vi "BASE-Main.vi"() -> ()   [LabVIEW 2017]
uses:
  <vilib>/Utility/error.llb/DialogType.ctl
  55ed0eea-cd20-493f-8468-85b8c1a0a0c0.vi
  Global/PLC_to_Auto.vi
panel:
  in  "AUTO":bool
  in  "PLAN EDITOR":bool
  in  "UNLOAD":bool
  in  "PLAN CREATOR":bool
  in  "i/o MANUAL":bool
  in  "i/o SCREEN":bool
  in  "HARDWARE SETTING":bool
  out "Status Number":i32
  out "Status":i32(ring)=1 items=["Stopped"=1, "StartPending"=2, "StopPending"=3, "Running"=4, "ContinuePending"=5, "PausePending"=6, "Paused"=7]
  in  "RECIPE":bool
  out "error out":errorcluster
  in  "Logout":bool
  in  "Stop":bool
  in  "Create Login":bool
  in  "Reports":bool
  in  "FEED":bool
  out "Time":string
  out "Date":string
  in  "Login":bool
  # "KITTING STATION"
types:
  T1 = enum8{"Enabled", "Disabled", "Disabled and Grayed Out"}
  T2 = typedef "DialogType.ctl" = u16
  T3 = enum32{"Invalid", "Standard", "Closed", "Hidden", "Minimized", "Maximized"}
  T4 = enum32{"invalid app kind", "Development System", "Run Time System", "Student Edition", "Embedded LabVIEW", "Evaluation", "Custom"}
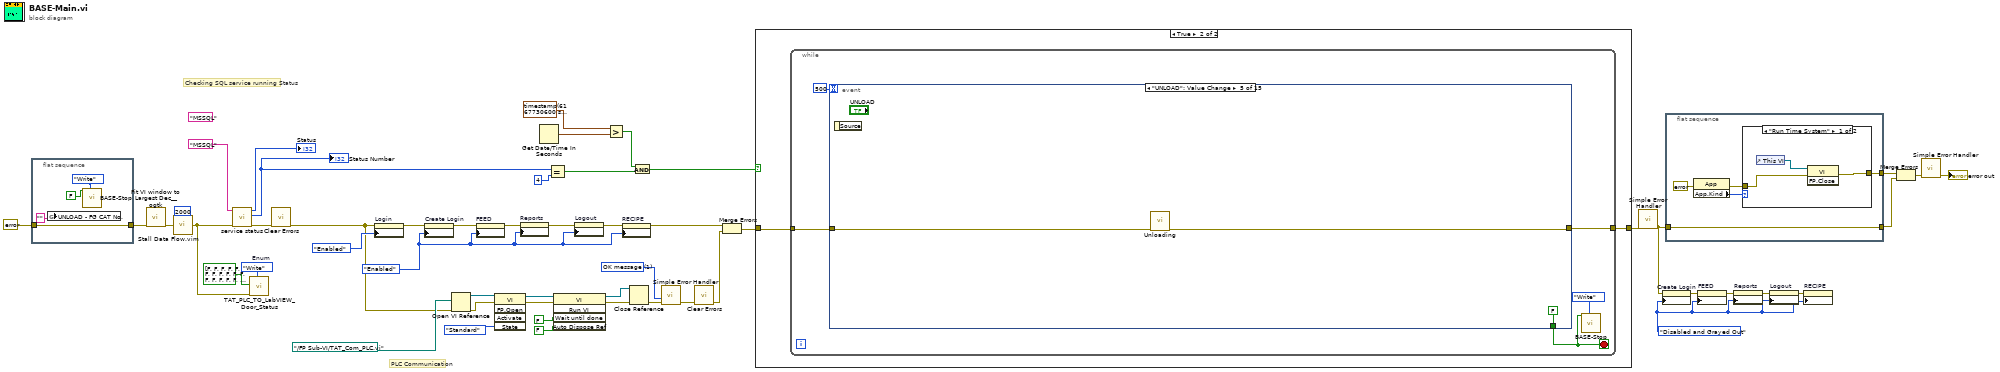
[diagram p0: block diagram]
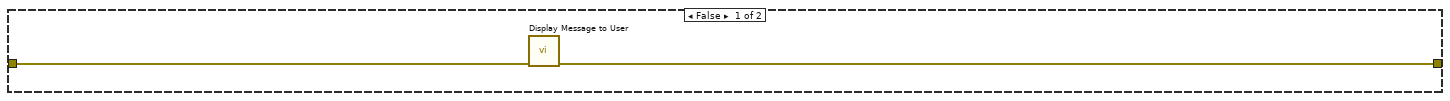
[diagram p3: hidden frame]
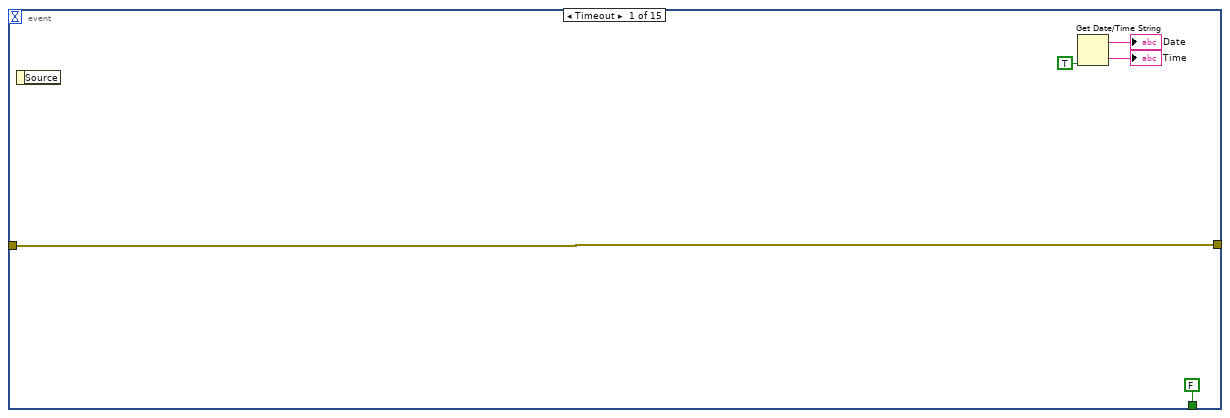
[diagram p4: hidden frame]
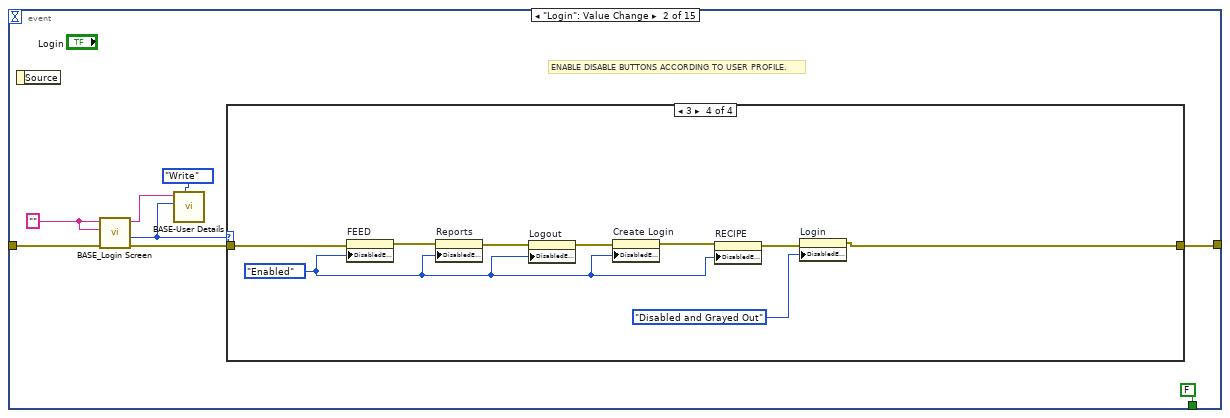
[diagram p5: hidden frame]
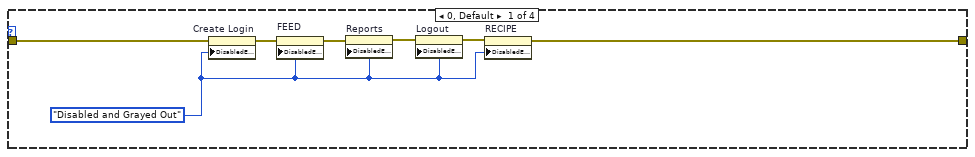
[diagram p6: hidden frame]
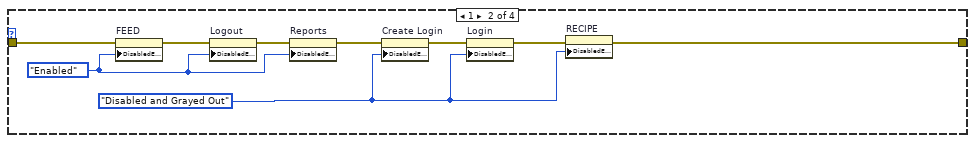
[diagram p7: hidden frame]
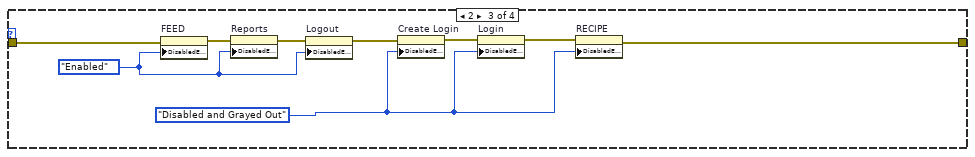
[diagram p8: hidden frame]
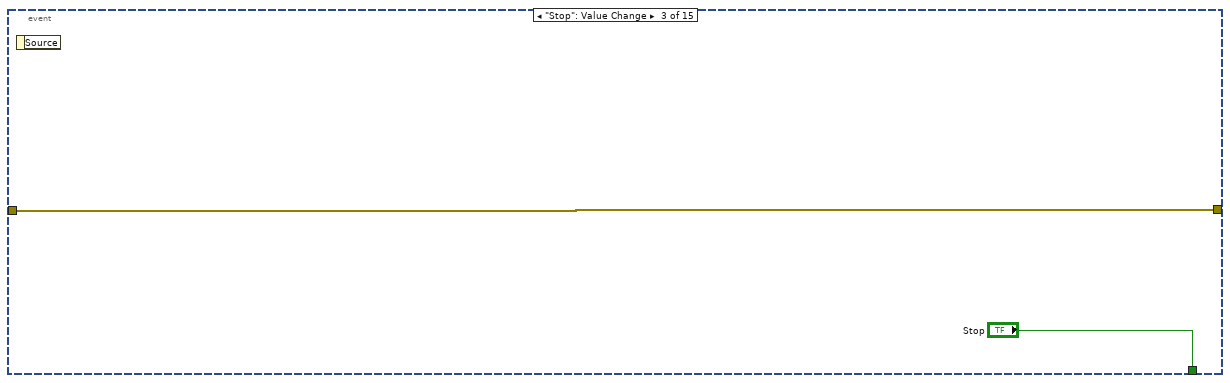
[diagram p9: hidden frame]
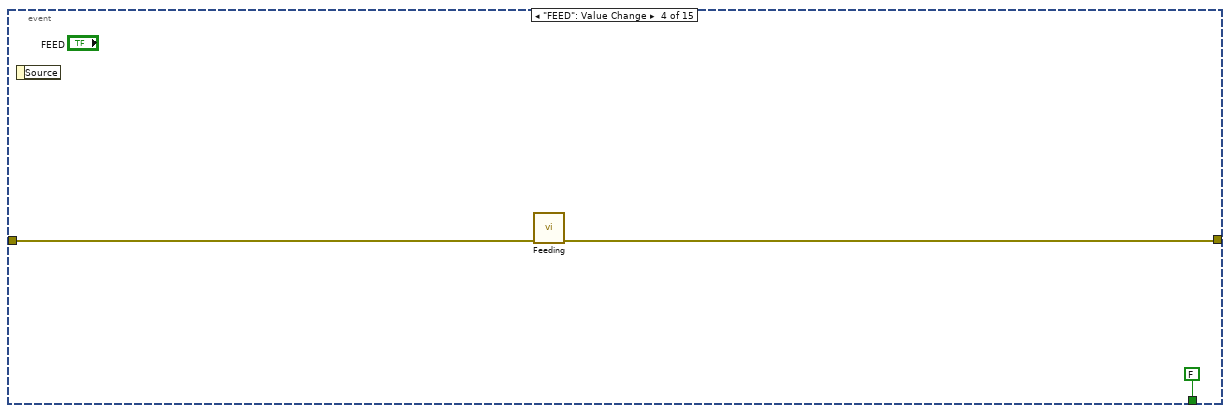
[diagram p10: hidden frame]
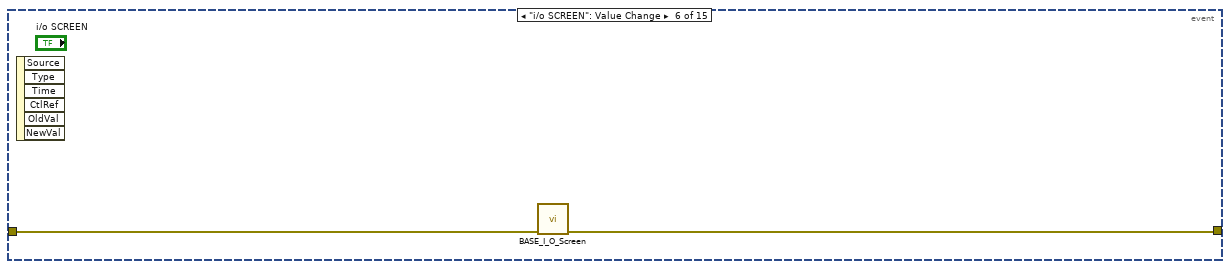
[diagram p11: hidden frame]
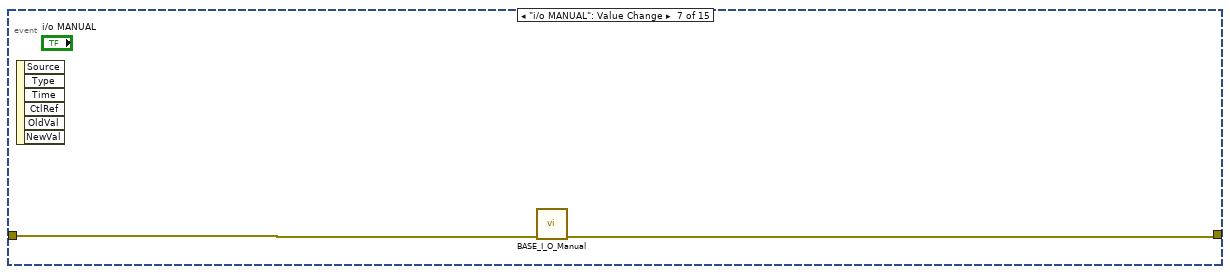
[diagram p12: hidden frame]
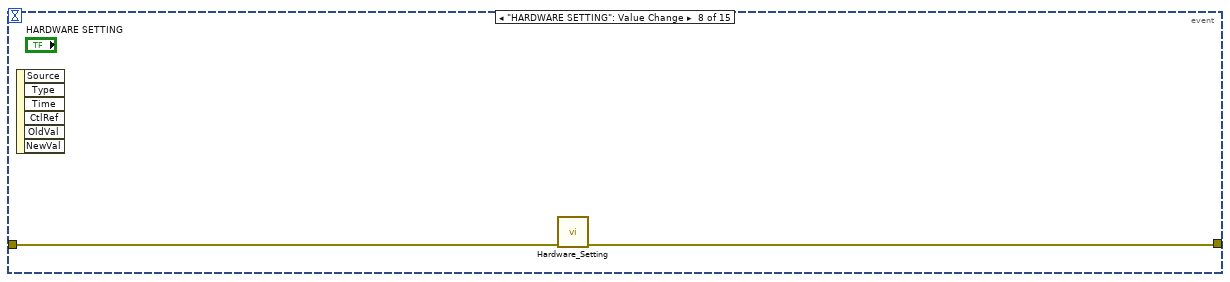
[diagram p13: hidden frame]
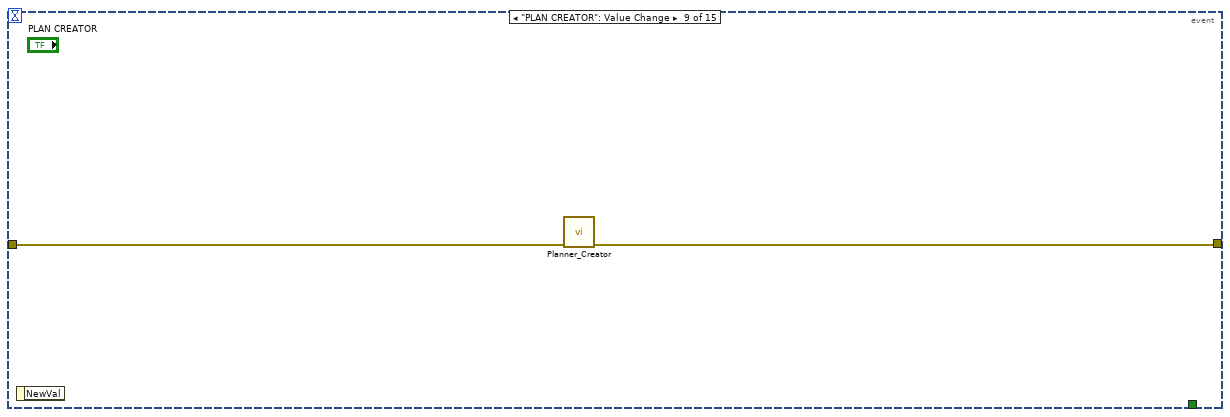
[diagram p14: hidden frame]
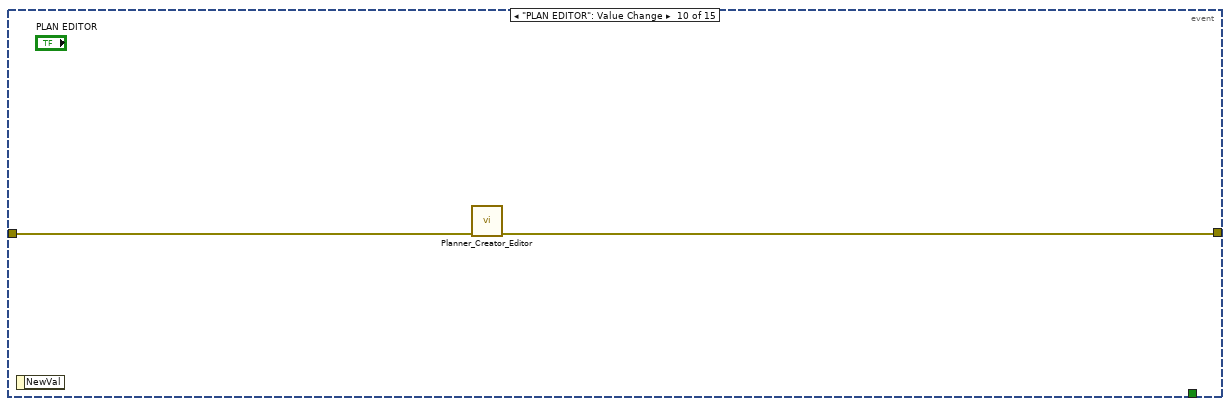
[diagram p15: hidden frame]
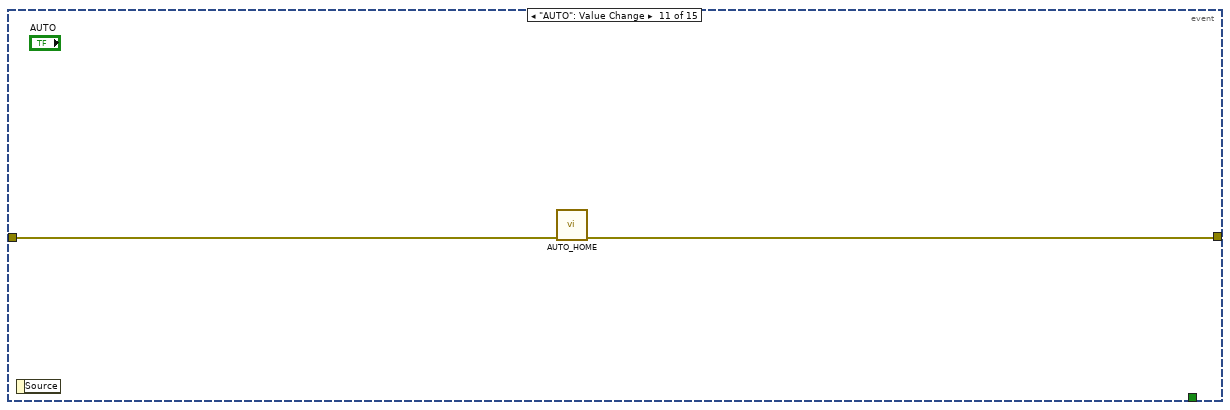
[diagram p16: hidden frame]
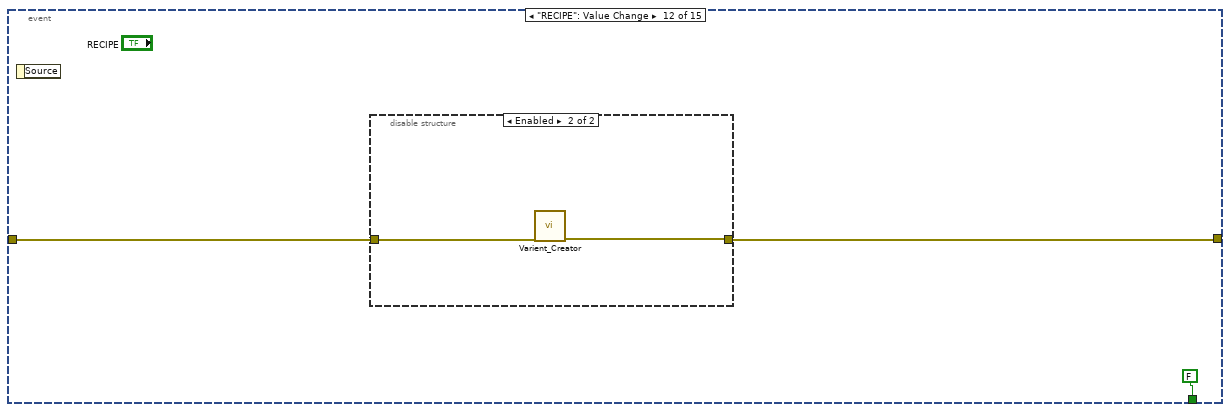
[diagram p17: hidden frame]
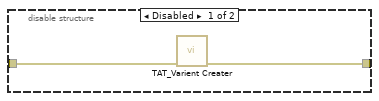
[diagram p18: hidden frame]
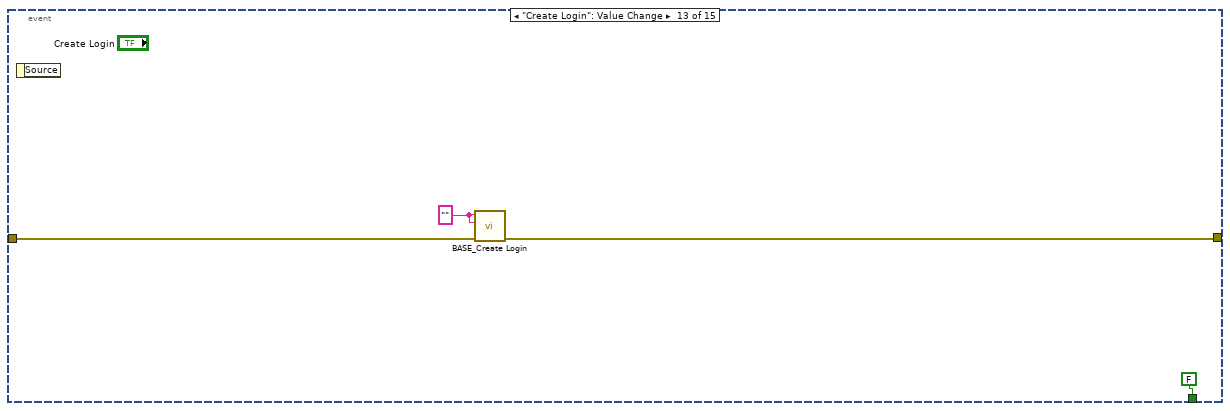
[diagram p19: hidden frame]
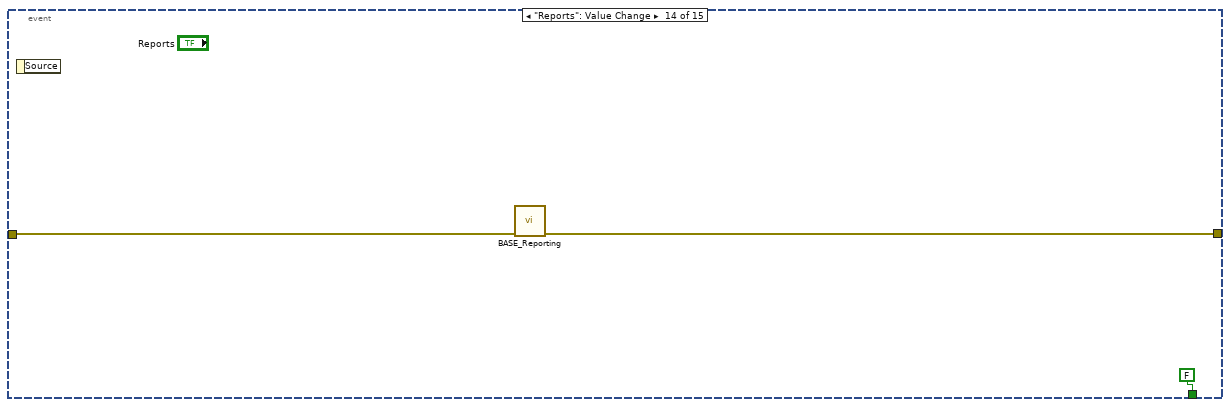
[diagram p20: hidden frame]
diagram:
  w3 = enum16{"Read", "Write"}."Write"  # Enum
  w10 = T1."Disabled and Grayed Out" ("Disabled")
  (unwired) "MSSQL" ("Service Name")
  w30 = T2 1 items=["no dialog", "OK message", "continue or stop message", "OK message + warnings", "continue/stop + warnings"] ("type of dialog (OK msg:1)")
  w11 = T1."Enabled" ("Disabled")
  # "PLC Communication"
  # "Checking SQL service running Status"
  n1 = flat-sequence {
    tunnel: [w56] -> w43
    tunnel: errorcluster {"status"=FALSE, "code"=0, "source"=""} ("error constant") -> [w56]
    frame #0 {
      n2 = global write "PLC_to_Auto.vi" "UNLOAD - FG CAT No."("") -> ()
      n3 = call "BASE-Stop.vi"("Enum"=enum16{"Read", "Write"}."Write", "Stop"=FALSE) -> ()  [unwired: 9 in, 1 out]
    }
  }
  n4 = call <userlib>:"Fit VI window to Largest Dec__ogtk.vi"("error in (no error)"=w43) -> ("error out"=w15:errorcluster)  [unwired: 5 in, 1 out]
  n5 = call "Stall Data Flow.vim"("value in"=w15, "milliseconds to wait"=u32 2000) -> ("value out"=w1:errorcluster)  [unwired: 1 out]
  n6 = call "service status.vi"("error in"=w1, "Service Name"="MSSQL") -> ("error out"=w22:errorcluster, "Status Number"=w24:i32, "Status"=→"Status":i32)  [unwired: 6 in, 1 out]
  "Status Number" <- w24
  n7 = call "TAT_PLC_TO_LabVIEW_Door_Status.vi"("Enum"=w3, "error in (no error)"=w1, "Array"=bool[] [FALSE, FALSE, FALSE, FALSE, FALSE, FALSE, FALSE, FALSE, FALSE, FALSE, FALSE, FALSE, FALSE, FALSE, FALSE, FALSE, FALSE, FALSE, FALSE, FALSE, FALSE, FALSE, FALSE, FALSE, FALSE, FALSE, FALSE]) -> ()  [unwired: 7 in, 2 out]
  n8 = call <vilib>:"Clear Errors.vi"("error in (no error)"=w22) -> ("error out"=w21:errorcluster)  [unwired: 5 in, 1 out]
  n9 = property on="Login" class="Bool"(error in=w21, "DisabledEnum"=T1."Enabled" ("Disabled")) -> (error out=w47:errorcluster)  [unwired: 1 in, 1 out]
  n10 = property on="Create Login" class="Bool"(error in=w47, "DisabledEnum"=w11) -> (error out=w51:errorcluster)  [unwired: 1 in, 1 out]
  n11 = Open VI Reference(vi path=path "../FP Sub-VI/TAT_Com_PLC.vi", error in (no error)=w21) -> (vi reference=w39:refnum<vi>, error out=w40:errorcluster)  [unwired: 4 in]
  n12 = property on="FEED" class="Bool"(error in=w51, "DisabledEnum"=w11) -> (error out=w12:errorcluster)  [unwired: 1 in, 1 out]
  n13 = invoke class="VI" method="FP.Open"(reference=w39, error in=w40, "State"=T3."Standard") -> (reference out=w42:refnum<vi>, error out=w41:errorcluster)  [unwired: 2 in, 3 out]
  n14 = property on="Reports" class="Bool"(error in=w12, "DisabledEnum"=w11) -> (error out=w45:errorcluster)  [unwired: 1 in, 1 out]
  n15 = Get Date/Time In Seconds() -> (seconds since 1Jan1904=w17:timestamp)
  n16 = Equal?(x=w24, y=4) -> (x = y?=w20:bool)
  n17 = invoke class="VI" method="Run VI"(reference=w42, error in=w41, "Wait until done"=FALSE ("Wait Until Done"), "Auto Dispose Ref"=FALSE ("Auto Dispose Reference")) -> (reference out=w38:refnum<vi>, error out=w37:errorcluster)  [unwired: 1 in, 3 out]
  n18 = property on="Logout" class="Bool"(error in=w45, "DisabledEnum"=w11) -> (error out=w13:errorcluster)  [unwired: 1 in, 1 out]
  n19 = Greater?(x=timestamp(6167730600 s since 1904-01-01), y=w17) -> (0:w16:bool)
  n20 = property on="RECIPE" class="Bool"(error in=w13, "DisabledEnum"=w11) -> (error out=w4:errorcluster)  [unwired: 1 in, 1 out]
  n21 = Close Reference(reference=w38, error in (no error)=w37) -> (error out=w31:errorcluster)
  n22 = And(x=w16, y=w20) -> (x .and. y?=w19:bool)
  n23 = call <vilib>:"Simple Error Handler.vi"("type of dialog (OK msg:1)"=w30, "error in (no error)"=w31) -> ("error out"=w29:errorcluster)  [unwired: 3 in, 4 out]
  n24 = call <vilib>:"Clear Errors.vi"("error in (no error)"=w29) -> ("error out"=w28:errorcluster)  [unwired: 5 in, 1 out]
  n25 = Merge Errors(w4, w28) -> (w33:errorcluster)
  n26 = case shown="True" w19 {
    tunnel: w33 -> [w58 w60]
    tunnel: [w57 w59] -> w52
    frame False {
      n27 = call "Display Message to User"("error in (no error)"=w58) -> ("error out"=w57:errorcluster)  [unwired: 9 in, 1 out]
    }
    frame True {
      n28 = while {
        tunnel: w60 -> [w64]
        tunnel: [w63] -> w59
        stop <- w61 stop-if-true
        n29 = event shown="[4] \"UNLOAD\": Value Change" {
          selector: _ -> [_ _ _ _ _ _ _ _ _ _ _ _ _ _ _]
          dyn-events: _ -> [_ _ _ _ _ _ _ _ _ _ _ _ _ _ _]
          timeout: 500 -> [_ _ _ _ _ _ _ _ _ _ _ _ _ _ _]
          tunnel: w64 -> [w68 w78 w113 w116 w119 w122 w124 w126 w128 w130 w132 w134 w143 w145 w153]
          tunnel: [w68 w71 w113 w115 w118 w121 w123 w125 w127 w129 w131 w133 w142 w144 w154] -> w63
          tunnel: [FALSE ("Stop") FALSE ("Stop") "Stop" FALSE ("Stop") FALSE ("Stop") _ _ _ _ _ _ FALSE ("Stop") FALSE ("Stop") FALSE ("Stop") FALSE ("Stop")] -> w61
          event Timeout {
            n30 = event-data() -> ()  [unwired: 1 in, 1 out]
            n31 = Get Date/Time String(want seconds? (F)=TRUE) -> (date string=→"Date":string, time string=→"Time":string)  [unwired: 2 in]
          }
          event "Login": Value Change {
            w74 = "" ("User Name")
            # "ENABLE DISABLE BUTTONS ACCORDING TO USER PROFILE."
            n32 = event-data() -> ()  [unwired: 1 in, 1 out]
            n33 = call "BASE_Login Screen.vi"("Error In"=w78, "Password"=w74, "User Name"=w74) -> ("error out"=w77:errorcluster, "Level"=w72:i32, "User Name Out"=w75:string)  [unwired: 5 in, 1 out]
            n34 = call "BASE-User Details.vi"("Enum"=enum16{"Read", "Write"}."Write", "Level In"=w72, "User Name In"=w75) -> ()  [unwired: 7 in, 2 out]
            n35 = case shown="3" w72 {
              tunnel: w77 -> [w83 w94 w103 w112]
              tunnel: [w79 w86 w95 w104] -> w71
              frame 0, Default {
                w80 = T1."Disabled and Grayed Out" ("Disabled")
                n36 = property on="Create Login" class="Bool"(error in=w83, "DisabledEnum"=w80) -> (error out=w85:errorcluster)  [unwired: 1 in, 1 out]
                n37 = property on="FEED" class="Bool"(error in=w85, "DisabledEnum"=w80) -> (error out=w84:errorcluster)  [unwired: 1 in, 1 out]
                n38 = property on="Reports" class="Bool"(error in=w84, "DisabledEnum"=w80) -> (error out=w81:errorcluster)  [unwired: 1 in, 1 out]
                n39 = property on="Logout" class="Bool"(error in=w81, "DisabledEnum"=w80) -> (error out=w82:errorcluster)  [unwired: 1 in, 1 out]
                n40 = property on="RECIPE" class="Bool"(error in=w82, "DisabledEnum"=w80) -> (error out=w79:errorcluster)  [unwired: 1 in, 1 out]
              }
              frame 1 {
                w88 = T1."Disabled and Grayed Out" ("Disabled")
                w87 = T1."Enabled" ("Disabled")
                n41 = property on="FEED" class="Bool"(error in=w94, "DisabledEnum"=w87) -> (error out=w90:errorcluster)  [unwired: 1 in, 1 out]
                n42 = property on="Logout" class="Bool"(error in=w90, "DisabledEnum"=w87) -> (error out=w92:errorcluster)  [unwired: 1 in, 1 out]
                n43 = property on="Reports" class="Bool"(error in=w92, "DisabledEnum"=w87) -> (error out=w93:errorcluster)  [unwired: 1 in, 1 out]
                n44 = property on="Create Login" class="Bool"(error in=w93, "DisabledEnum"=w88) -> (error out=w91:errorcluster)  [unwired: 1 in, 1 out]
                n45 = property on="Login" class="Bool"(error in=w91, "DisabledEnum"=w88) -> (error out=w89:errorcluster)  [unwired: 1 in, 1 out]
                n46 = property on="RECIPE" class="Bool"(error in=w89, "DisabledEnum"=w88) -> (error out=w86:errorcluster)  [unwired: 1 in, 1 out]
              }
              frame 2 {
                w96 = T1."Disabled and Grayed Out" ("Disabled")
                w97 = T1."Enabled" ("Disabled")
                n47 = property on="FEED" class="Bool"(error in=w103, "DisabledEnum"=w97) -> (error out=w100:errorcluster)  [unwired: 1 in, 1 out]
                n48 = property on="Reports" class="Bool"(error in=w100, "DisabledEnum"=w97) -> (error out=w102:errorcluster)  [unwired: 1 in, 1 out]
                n49 = property on="Logout" class="Bool"(error in=w102, "DisabledEnum"=w97) -> (error out=w98:errorcluster)  [unwired: 1 in, 1 out]
                n50 = property on="Create Login" class="Bool"(error in=w98, "DisabledEnum"=w96) -> (error out=w101:errorcluster)  [unwired: 1 in, 1 out]
                n51 = property on="Login" class="Bool"(error in=w101, "DisabledEnum"=w96) -> (error out=w99:errorcluster)  [unwired: 1 in, 1 out]
                n52 = property on="RECIPE" class="Bool"(error in=w99, "DisabledEnum"=w96) -> (error out=w95:errorcluster)  [unwired: 1 in, 1 out]
              }
              frame 3 {
                w105 = T1."Enabled" ("Disabled")
                n53 = property on="FEED" class="Bool"(error in=w112, "DisabledEnum"=w105) -> (error out=w107:errorcluster)  [unwired: 1 in, 1 out]
                n54 = property on="Reports" class="Bool"(error in=w107, "DisabledEnum"=w105) -> (error out=w111:errorcluster)  [unwired: 1 in, 1 out]
                n55 = property on="Logout" class="Bool"(error in=w111, "DisabledEnum"=w105) -> (error out=w110:errorcluster)  [unwired: 1 in, 1 out]
                n56 = property on="Create Login" class="Bool"(error in=w110, "DisabledEnum"=w105) -> (error out=w109:errorcluster)  [unwired: 1 in, 1 out]
                n57 = property on="RECIPE" class="Bool"(error in=w109, "DisabledEnum"=w105) -> (error out=w108:errorcluster)  [unwired: 1 in, 1 out]
                n58 = property on="Login" class="Bool"(error in=w108, "DisabledEnum"=T1."Disabled and Grayed Out" ("Disabled")) -> (error out=w104:errorcluster)  [unwired: 1 in, 1 out]
              }
            }
          }
          event "Stop": Value Change {
            n59 = event-data() -> ()  [unwired: 1 in, 1 out]
          }
          event "FEED": Value Change {
            n60 = event-data() -> ()  [unwired: 1 in, 1 out]
            n61 = call "Feeding.vi"("error In"=w116) -> ("error out"=w115:errorcluster)  [unwired: 10 in]
          }
          event "UNLOAD": Value Change {
            n62 = event-data() -> ()  [unwired: 1 in, 1 out]
            n63 = call "Unloading.vi"("error In"=w119) -> ("error out"=w118:errorcluster)  [unwired: 10 in]
          }
          event "i/o SCREEN": Value Change {
            n64 = event-data() -> ()  [unwired: 1 in, 6 out]
            n65 = call "BASE_I_O_Screen.vi"("error in (no error)"=w122) -> ("error out"=w121:errorcluster)  [unwired: 10 in]
          }
          event "i/o MANUAL": Value Change {
            n66 = event-data() -> ()  [unwired: 1 in, 6 out]
            n67 = call "BASE_I_O_Manual.vi"("error in (no error)"=w124) -> ("error out"=w123:errorcluster)  [unwired: 10 in]
          }
          event "HARDWARE SETTING": Value Change {
            n68 = event-data() -> ()  [unwired: 1 in, 6 out]
            n69 = call "Hardware_Setting.vi"("Error in"=w126) -> ("error out 2"=w125:errorcluster)  [unwired: 10 in]
          }
          event "PLAN CREATOR": Value Change {
            n70 = event-data() -> ()  [unwired: 1 in, 1 out]
            n71 = call "Planner_Creator.vi"("error in (no error)"=w128) -> ("error out"=w127:errorcluster)  [unwired: 10 in]
          }
          event "PLAN EDITOR": Value Change {
            n72 = event-data() -> ()  [unwired: 1 in, 1 out]
            n73 = call "Planner_Creator_Editor.vi"("error in (no error)"=w130) -> ("error out"=w129:errorcluster)  [unwired: 10 in]
          }
          event "AUTO": Value Change {
            n74 = event-data() -> ()  [unwired: 1 in, 1 out]
            n75 = call "AUTO_HOME.vi"("error in (no error)"=w132) -> ("error out"=w131:errorcluster)  [unwired: 10 in]
          }
          event "RECIPE": Value Change {
            n76 = event-data() -> ()  [unwired: 1 in, 1 out]
            n77 = disable-structure shown="Enabled" {
              disable-tunnel: w134 -> [w137 w139]
              disable-tunnel: [w136 w138] -> w133
              frame Disabled {
                n78 = call "TAT_Varient Creater.vi"("error in (no error)"=w137) -> ("error out"=w136:errorcluster)  [unwired: 10 in]
              }
              frame Enabled {
                n79 = call "Varient_Creator.vi"("error in (no error)"=w139) -> ("error out"=w138:errorcluster)  [unwired: 10 in]
              }
            }
          }
          event "Create Login": Value Change {
            w141 = "" ("User Name")
            n80 = event-data() -> ()  [unwired: 1 in, 1 out]
            n81 = call "BASE_Create Login.vi"("Error In"=w143, "Password"=w141, "User Name"=w141) -> ("error out"=w142:errorcluster)  [unwired: 6 in]
          }
          event "Reports": Value Change {
            n82 = event-data() -> ()  [unwired: 1 in, 1 out]
            n83 = call "BASE_Reporting.vi"("error in (no error)"=w145) -> ("error out"=w144:errorcluster)  [unwired: 10 in]
          }
          event "Logout": Value Change {
            w148 = T1."Disabled and Grayed Out" ("Disabled")
            n84 = event-data() -> ()  [unwired: 1 in, 1 out]
            n85 = property on="Logout" class="Bool"(error in=w153, "DisabledEnum"=w148) -> (error out=w149:errorcluster)  [unwired: 1 in, 1 out]
            n86 = property on="Create Login" class="Bool"(error in=w149, "DisabledEnum"=w148) -> (error out=w156:errorcluster)  [unwired: 1 in, 1 out]
            n87 = property on="FEED" class="Bool"(error in=w156, "DisabledEnum"=w148) -> (error out=w155:errorcluster)  [unwired: 1 in, 1 out]
            n88 = property on="Reports" class="Bool"(error in=w155, "DisabledEnum"=w148) -> (error out=w150:errorcluster)  [unwired: 1 in, 1 out]
            n89 = property on="RECIPE" class="Bool"(error in=w150, "DisabledEnum"=w148) -> (error out=w147:errorcluster)  [unwired: 1 in, 1 out]
            n90 = property on="Login" class="Bool"(error in=w147, "DisabledEnum"=T1."Enabled" ("Disabled")) -> (error out=w154:errorcluster)  [unwired: 1 in, 1 out]
          }
        }
        n91 = call "BASE-Stop.vi"("Enum"=enum16{"Read", "Write"}."Write", "Stop"=w61) -> ()  [unwired: 9 in, 1 out]
      }
    }
  }
  n92 = call <vilib>:"Simple Error Handler.vi"("error in (no error)"=w52) -> ("error out"=w5:errorcluster)  [unwired: 4 in, 4 out]
  n93 = property on="Create Login" class="Bool"(error in=w5, "DisabledEnum"=w10) -> (error out=w6:errorcluster)  [unwired: 1 in, 1 out]
  n94 = flat-sequence {
    tunnel: [w158] -> w50
    tunnel: [w157] -> w48
    tunnel: w5 -> [w157]
    frame #0 {
      n95 = property class="App"(error in=errorcluster {"status"=FALSE, "code"=0, "source"=""} ("error in (no error)")) -> (error out=w160:errorcluster, "App.Kind"=w161:T4)  [unwired: 1 in, 1 out]
      n96 = case shown="\"Run Time System\"" w161 {
        tunnel: w160 -> [w163 w165]
        tunnel: [w162 w165] -> w158
        frame "Run Time System" {
          n97 = control-ref of="This VI"() -> (w164:refnum<vi>)
          n98 = invoke class="VI" method="FP.Close"(reference=w164, error in=w163) -> (error out=w162:errorcluster)  [unwired: 1 in, 2 out]
        }
        frame "Development System", Default {
        }
      }
    }
  }
  n99 = property on="FEED" class="Bool"(error in=w6, "DisabledEnum"=w10) -> (error out=w9:errorcluster)  [unwired: 1 in, 1 out]
  n100 = property on="Reports" class="Bool"(error in=w9, "DisabledEnum"=w10) -> (error out=w7:errorcluster)  [unwired: 1 in, 1 out]
  n101 = property on="Logout" class="Bool"(error in=w7, "DisabledEnum"=w10) -> (error out=w8:errorcluster)  [unwired: 1 in, 1 out]
  n102 = property on="RECIPE" class="Bool"(error in=w8, "DisabledEnum"=w10) -> ()  [unwired: 1 in, 2 out]
  n103 = Merge Errors(w50, w48) -> (w49:errorcluster)
  n104 = call <vilib>:"Simple Error Handler.vi"("error in (no error)"=w49) -> ("error out"=→"error out":errorcluster)  [unwired: 4 in, 4 out]
